vi "Create Channel Array.vi"(8 "error in":errorcluster, 10 "channel settings":T1[](array[typedef]), 11 "PWM mode in":refnum<class "PWM Mode.lvclass">) -> (0 "error out":errorcluster, 2 "channels":refnum<class "PWM Output Channel.lvclass">[](array[class]), 3 "PWM mode out":refnum<class "PWM Mode.lvclass">)   [LabVIEW 2020, in "Scan Engine Scripting.lvlib" / "PWM Mode.lvclass"]
uses:
  PWM Mode.lvclass
  Controls/pwm channel settings.ctl
  Channel Classes/PWM Output Channel/Frequency.ctl
  Channel Classes/PWM Output Channel/PWM Output Channel.lvclass
  Scan Engine Scripting.lvlib
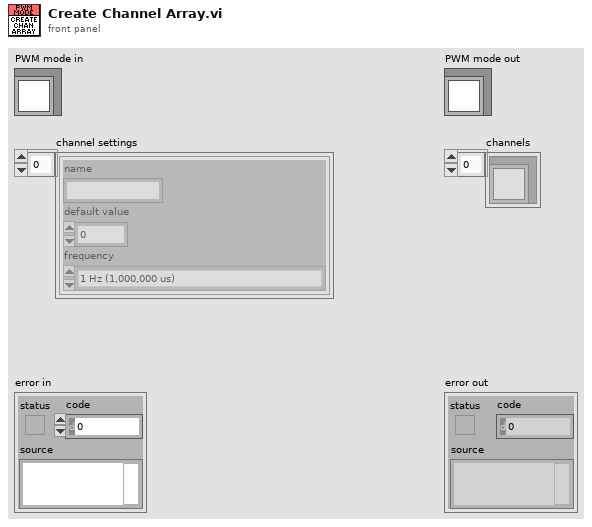
[diagram p1: front panel]
types:
  T1 = typedef "Scan Engine Scripting.lvlib/pwm channel settings.ctl" = cluster{"name":string, "default value":dbl, "frequency":T2}
  T2 = typedef "Scan Engine Scripting.lvlib/PWM Output Channel.lvclass/Frequency.ctl" = enum16{"1 Hz (1,000,000 us)", "50 Hz (20,000 us)", "250 Hz (4,000 us)", "500 Hz (2,000 us)", "1 kHz (1,000 us)", "5 kHz (200 us)", "10 kHz (100 us)", "20 kHz (50 us)"}
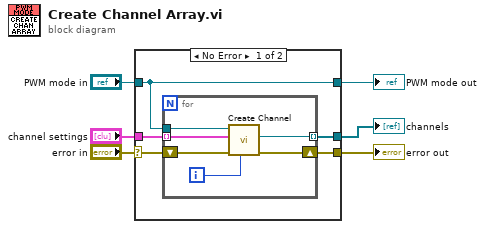
[diagram p0: block diagram]
diagram:
  n1 = case shown="No Error" "error in" {
    selector: "error in" -> [w9 w19]
    tunnel: [w8 w19] -> w5
    tunnel: [w11 w18] -> w3
    tunnel: "PWM mode in" -> [w11 w18]
    tunnel: "channel settings" -> [w10 _]
    tunnel: [w7 _] -> w1
    frame No Error {
      n2 = for {
        tunnel: w10 -> [w12] mode=indexing
        shift-right: [w16] -> w8
        shift-left: w9 -> [w17]
        tunnel: w11 -> [w14]
        tunnel: [w15] -> w7 mode=indexing
        i -> [w13]
        n3 = call "Create Channel.vi"("index"=w13, "error in"=w17, "channel settings"=w12, "PWM mode in"=w14) -> ("error out"=w16:errorcluster, "PWM channel"=w15:refnum<class "PWM Output Channel.lvclass">)  [unwired: 5 in, 1 out]
      }
    }
    frame Error {
    }
  }
  "error out" <- w5
  "PWM mode out" <- w3
  "channels" <- w1
